vi "Alazar_SetTriggerDelay - ATS-SDK.vi"(8 "error in (no error)":errorcluster, 10 "Delay in Pts":u32, 11 "Handle":u32) -> (0 "error out":errorcluster, 1 "Return Code":u32, 3 "Handle Out":u32)   [LabVIEW 2022 SP3]
doc: "_____AlazarTech, Scope_____\n\nSet the Trigger delay"
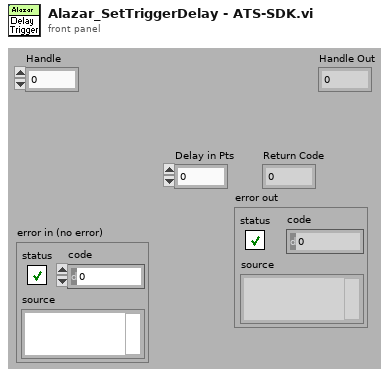
[diagram p1: front panel]
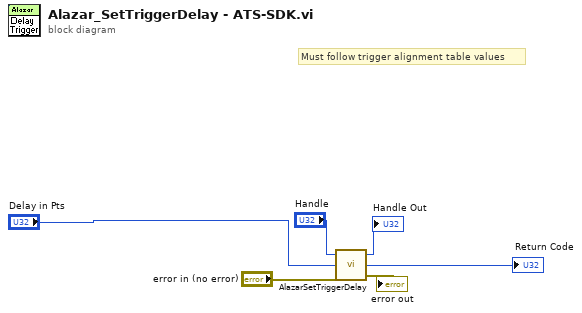
[diagram p0: block diagram]
diagram:
  # "Must follow trigger alignment table values"
  n1 = call "AlazarSetTriggerDelay.vi"("error in (no error)"="error in (no error)", "Delay"="Delay in Pts", "Handle"="Handle") -> ("error out"=→"error out":errorcluster, "Return Code"=→"Return Code":u32, "Handle"=→"Handle Out":u64)
